vi "HFRR ADV v07 new software.vi"() -> ()   [LabVIEW 2025] (continued)
            n3590 = Concatenate Strings(w4524, w4494) -> (w4555:string)
            n3591 = Concatenate Strings(w4576, w4474, w4577, w4570) -> (w4579:string)
            n3592 = Concatenate Strings(w4526, w4521) -> (w4553:string)
            n3593 = Concatenate Strings(w4525, w4511) -> (w4552:string)
            n3594 = Concatenate Strings(w4524, w4493) -> (w4554:string)
            n3595 = Concatenate Strings(w4526, w4520) -> (w4548:string)
            n3596 = Concatenate Strings(w4525, w4510) -> (w4549:string)
            n3597 = Concatenate Strings(w4524, w4492) -> (w4547:string)
            n3598 = Concatenate Strings(w4526, w4519) -> (w4545:string)
            n3599 = Concatenate Strings(w4525, w4509) -> (w4544:string)
            n3600 = Concatenate Strings(w4524, w4491) -> (w4546:string)
            n3601 = Concatenate Strings(w4556, w4557, w4555) -> (w4558:string)
            n3602 = Concatenate Strings(w4526, w4518) -> (w4535:string)
            n3603 = Concatenate Strings(w4525, w4508) -> (w4536:string)
            n3604 = Concatenate Strings(w4526, w4517) -> (w4532:string)
            n3605 = Concatenate Strings(w4525, w4507) -> (w4531:string)
            n3606 = Concatenate Strings(w4524, w4490) -> (w4534:string)
            n3607 = Concatenate Strings(w4524, w4489) -> (w4533:string)
            n3608 = Concatenate Strings("{\"SecretKey\":\"", w4573, w4579, "\",\"UUID\" : \"", w4568, "\",\"SensorInformation\":", "[{" ("string")) -> (w4506:string)
            n3609 = Concatenate Strings(w4553, w4552, w4554) -> (w4551:string)
            n3610 = Concatenate Strings(w4548, w4549, w4547) -> (w4550:string)
            n3611 = Concatenate Strings(w4545, w4544, w4546) -> (w4543:string)
            n3612 = Concatenate Strings(w4535, w4536, w4534) -> (w4537:string)
            n3613 = Concatenate Strings(w4532, w4531, w4533) -> (w4530:string)
            n3614 = Concatenate Strings(w4529, w4541, w4558, w4499) -> (w4505:string)
            n3615 = Concatenate Strings(w4529, w4540, w4551, w4499) -> (w4504:string)
            n3616 = Concatenate Strings(w4529, w4539, w4550, w4499) -> (w4503:string)
            n3617 = Concatenate Strings(w4529, w4538, w4543, w4499) -> (w4502:string)
            n3618 = Concatenate Strings(w4529, w4528, w4537, w4499) -> (w4501:string)
            n3619 = Concatenate Strings(w4529, w4527, w4530, "\"}" ("string")) -> (w4500:string)
            n3620 = Concatenate Strings(w4506, w4505, w4504, w4503, w4502, w4501, w4500, "]}" ("string")) -> (w4497:string)
            n3621 = local read "SEN.RUN HRS"() -> (w4464:dbl)
            n3622 = disable-structure shown="Disabled" {
              frame Disabled {
                n3623 = local read "state"() -> (w4583:string[])
                n3624 = Delete From Array(array=w4583, index=0) -> (array with subset deleted=w4581:string[])  [unwired: 1 in, 1 out]
                n3625 = for {
                  N: 6 -> [_]
                  tunnel: w4581 -> [w4594] mode=indexing
                  tunnel: [w4593] -> w4580 mode=indexing
                  n3626 = Equal?(x=w4594, y="Warning") -> (x = y?=w4590:bool)
                  n3627 = Equal?(x=w4594, y="Healthy") -> (x = y?=w4587:bool)
                  n3628 = Select(t="2" ("y"), s=w4590, f="3" ("y")) -> (s? t:f=w4585:string)
                  n3629 = Select(t="1" ("y"), s=w4587, f=w4585) -> (s? t:f=w4593:string)
                }
                "state1" <- w4580
              }
              frame Enabled {
              }
            }
            n3630 = stacked-sequence {
              tunnel: w4497 -> [w4605 _ _]
              tunnel: [_ _ w4621] -> _
              frame #0 {
                (unwired) FALSE ("convert eol (F)")
                w4607 = enum16{"start", "end", "current"}."start" ("pos mode (0:2)")
                n3631 = local read "Path"() -> (w4601:path)
                n3632 = Path To String(path=w4601) -> (string=w4613:string)
                n3633 = Concatenate Strings(w4613, "\\", "Sensor File Name") -> (w4614:string)
                n3634 = local write "standard output 2"(" ") -> ()
                n3635 = String To Path(string=w4614) -> (path=w4604:path)
                n3636 = call <vilib>:"Open_Create_Replace File.vi"("advisory dialog? (display:T)"=FALSE, "function (open:0)"=T29."create or replace", "file path"=w4604) -> ("error out"=w4617:errorcluster, "refnum"=w4616:refnum<file>)  [unwired: 5 in, 2 out]
                n3637 = Set File Position(refnum=w4616, from (0:start)=w4607, error in=w4617) -> (refnum out=w4597:refnum<file>, error out=w4596:errorcluster)  [unwired: 1 in]
                n3638 = Write to Binary File(file (use dialog)=w4597, data=" ", error in=w4596, 5:FALSE ("prepend array or string size? (T)")) -> (refnum out=w4608:refnum<file>, error out=w4609:errorcluster)  [unwired: 2 in, 1 out]
                n3639 = Set File Position(offset (in bytes) (0)=w4607, refnum=w4608, error in=w4609) -> (refnum out=w4600:refnum<file>, error out=w4599:errorcluster)  [unwired: 1 in]
                n3640 = Write to Binary File(file (use dialog)=w4600, data=w4605, error in=w4599, 5:FALSE ("prepend array or string size? (T)")) -> (error out=w4603:errorcluster)  [unwired: 2 in, 2 out]
                n3641 = flat-sequence {
                  tunnel: w4604 -> [w4619]
                  tunnel: w4603 -> [_]
                  frame #0 {
                    n3642 = call <vilib>:"Read Characters From File.vi"("file path (dialog if empty)"=w4619) -> ("character string"=→"Sensor Health JSON string":string)  [unwired: 5 in, 3 out]
                  }
                }
                "SinglePoint  2" <- w4605
              }
              frame #1 {
              }
              frame #2 {
                (unwired) "\"Stored\": true" ("string")
                n3643 = call <vilib>:"System Exec.vi"("run minimized? (F)"=TRUE, "wait until completion? (T)"=TRUE, "working directory"=path "C:/LAB-IQ-NXT", "command line"="C:\\LAB-IQ-NXT\\JPostH.bat") -> ("standard error"=→"Respose From Server 2":string, "standard output"=w4624:string)  [unwired: 4 in, 2 out]
                "standard output 2" <- w4624
                n3644 = Match Pattern(string=w4624, regular expression="JSONH Check String") -> (match substring=w4622:string, offset past match=w4621:i32)  [unwired: 1 in, 2 out]
                n3645 = Equal?(x=w4622, y="JSONH Check String") -> (x = y?=→"Upload \nConfirmed 2":bool)
              }
            }
            n3646 = Divide(x=w4464, y=3600.0 ("f")) -> (x/y=w4457:dbl)
            n3647 = local read "run time"() -> (w4514:string[])
            n3648 = Round To Nearest(number=w4457) -> (nearest integer value=w4456:dbl)
            n3649 = Number To Decimal String(number=w4456) -> (decimal integer string=w4455:string)  [unwired: 1 in]
            n3650 = Index Array(array="Sensor Information", index (col) #1=0 ("disabled index (col)"), index (col) #2=1 ("index (col)"), index (col) #3=2 ("index (col)"), index (col) #4=3 ("index (col)")) -> (element #1=→"Sensor name":string[], element #2=→"model num":string[], element #3=→"run time":string[], element #4=→"state":string[])  [unwired: 4 in]
            n3651 = Insert Into Array(array=w4514, index=1, new element #1=w4455, new element #2=w4455, new element #3=w4455, new element #4=w4455, new element #5=w4455, new element #6=w4455) -> (w4479:string[])
            "run" <- w4479
            n3652 = local read "out"() -> (w4461:string[])
            n3653 = local read "Sensor Information"() -> (w4481:string[][])
            n3654 = Replace Array Subset(array=w4481, new element #1=w4479, index (col) #1=2 ("disabled index (col)"), new element #2=w4461, index (col) #2=3 ("index (col)")) -> (w4480:string[][])  [unwired: 2 in]
            n3655 = local write "Sensor Information"(w4480) -> ()
          }
        }
        n3656 = case shown="True" w4428 {
          frame False {
          }
          frame True {
            n3657 = Equal?(x="FLAG", y=0.0) -> (x = y?=w4445:bool)
            n3658 = case shown="False" w4445 {
              frame False {
                n3659 = Get Date/Time In Seconds() -> (seconds since 1Jan1904=w4451:timestamp)
                n3660 = local read "START 2"() -> (w4449:dbl)
                n3661 = To Double Precision Float(number=w4451) -> (double precision float=w4450:dbl)
                n3662 = Subtract(x=w4450, y=w4449) -> (x-y=→"SENSOR TIME  2":dbl)
              }
              frame True {
                n3663 = Get Date/Time In Seconds() -> (seconds since 1Jan1904=w4453:timestamp)
                n3664 = To Double Precision Float(number=w4453) -> (double precision float=→"START 2":dbl)
                n3665 = local write "FLAG"(100.0 ("FLAG")) -> ()
              }
            }
          }
        }
        n3666 = disable-structure shown="Disabled" {
          disable-tunnel: w4431 -> [w4440 _]
          disable-tunnel: [w4439 _] -> w4430
          frame Disabled {
            n3667 = local read "Json St Flg"() -> (w4438:bool)
            n3668 = case shown="True" w4438 {
              tunnel: w4440 -> [w4441 w4443]
              tunnel: [w4441 w4442] -> w4439
              frame False {
              }
              frame True {
                n3669 = Increment(x=w4443) -> (x+1=w4442:dbl)
                "T cycle" <- w4442
                n3670 = local write "Json St Flg"(FALSE ("Json St Flg")) -> ()
              }
            }
          }
          frame Enabled {
          }
        }
        n3671 = local read "Quit"() -> (w4425:bool)
      }
    }
    frame Enabled {
    }
  }
  n3672 = stacked-sequence {
    tunnel: [w4823] -> w38
    frame #0 {
      w4823 = FALSE ("Upload \nConfirmed")
      n3673 = local write "Upload \nConfirmed"(w4823) -> ()
      n3674 = local write "St Str"("") -> ()
    }
  }
  n3675 = disable-structure shown="Disabled" {
    disable-tunnel: w38 -> [w4824 _]
    frame Disabled {
      n3676 = case shown="True" {
        selector: _ -> [_ _]
        tunnel: w4824 -> [_ w4825]
        frame False {
        }
        frame True {
          n3677 = while {
            tunnel: [w4831] -> _
            tunnel: w4825 -> [_]
            i -> [w4831]
            stop <- w4826 stop-if-true
            n3678 = local read "Json End Flg"() -> (w4830:bool)
            n3679 = Wait (ms)(milliseconds to wait=u32 20 ("Refresh Rate (ms)")) -> ()  [unwired: 1 out]
            n3680 = local read "refresh flag"() -> (w4827:bool)
            n3681 = local read "RUN"() -> (w4828:bool)
            n3682 = And(x=w4828, y=w4827) -> (x .and. y?=w4829:bool)
            n3683 = Or(x=w4829, y=w4830) -> (x .or. y?=w4832:bool)
            "AR Led" <- w4832
            n3684 = case shown="True" w4832 {
              frame False {
              }
              frame True {
                w4849 = "\",\""
                n3685 = local read "UUID"() -> (w4847:string)
                n3686 = local write "refresh flag"(FALSE ("refresh flag")) -> ()
                n3687 = local read "time"() -> (w4836:dbl)
                n3688 = Multiply(x=w4836, y=60.0) -> (x*y=w4835:dbl)
                n3689 = Concatenate Strings("UUID\" : \"", w4847, "\"}") -> (w4850:string)
                n3690 = Number To Fractional String(number=w4835, width (-)=i16 10, precision (6)=i16 4) -> (F-format string=w4864:string)  [unwired: 1 in]
                n3691 = Concatenate Strings("{", "\"Time\":\"", w4864, w4849) -> (w4859:string)
                n3692 = stacked-sequence {
                  tunnel: w4849 -> [w4912 w4920 w4927 w4935 w4943 w4952 w4959]
                  tunnel: [w4913 _ _ _ _ _ _] -> w4863
                  tunnel: [_ w4921 _ _ _ _ _] -> w4862
                  tunnel: [_ _ w4928 _ _ _ _] -> w4861
                  tunnel: [_ _ _ w4937 _ _ _] -> w4860
                  tunnel: w4850 -> [_ _ _ _ _ _ w4970]
                  tunnel: [_ _ _ _ _ _ w4969] -> w4846
                  tunnel: [_ _ _ _ _ w4949 _] -> w4845
                  tunnel: [_ _ _ _ w4942 _ _] -> w4844
                  frame #0 {
                    n3693 = local read "NORMAL LOAD"() -> (w4911:dbl)
                    n3694 = Number To Fractional String(number=w4911, width (-)=i16 10, precision (6)=i16 4) -> (F-format string=w4914:string)  [unwired: 1 in]
                    n3695 = Concatenate Strings("NormalLoad\":\"", w4914, w4912) -> (w4913:string)
                  }
                  frame #1 {
                    n3696 = local read "Temp"() -> (w4919:dbl)
                    n3697 = Number To Fractional String(number=w4919, width (-)=i16 10, precision (6)=i16 4) -> (F-format string=w4922:string)  [unwired: 1 in]
                    n3698 = Concatenate Strings("Temperature\":\"", w4922, w4920) -> (w4921:string)
                  }
                  frame #2 {
                    n3699 = local read "cof"() -> (w4925:dbl)
                    n3700 = Number To Fractional String(number=w4925, width (-)=i16 10, precision (6)=i16 4) -> (F-format string=w4929:string)  [unwired: 1 in]
                    n3701 = Concatenate Strings("FrictionalForce\":\"", w4929, w4927) -> (w4928:string)
                  }
                  frame #3 {
                    n3702 = local read "Set Hz"() -> (w4933:dbl)
                    n3703 = Multiply(x=w4933, y=60.0) -> (x*y=w4932:dbl)
                    n3704 = Number To Fractional String(number=w4932, width (-)=i16 10, precision (6)=i16 4) -> (F-format string=w4938:string)  [unwired: 1 in]
                    n3705 = Concatenate Strings("Speed\":\"", w4938, w4935) -> (w4937:string)
                  }
                  frame #4 {
                    n3706 = local read item#-1() -> (w4941)
                    n3707 = Number To Fractional String(number=w4941, width (-)=i16 10, precision (6)=i16 4) -> (F-format string=w4945:string)  [unwired: 1 in]
                    n3708 = Concatenate Strings("LinearDeformation\":\"", w4945, w4943) -> (w4942:string)
                  }
                  frame #5 {
                    n3709 = local read "AIR TEMP"() -> (w4948:dbl)
                    n3710 = local read "Json St Flg"() -> (w4950:bool)
                    n3711 = local read "Json End Flg"() -> (w4951:bool)
                    n3712 = Number To Fractional String(number=w4948, width (-)=i16 10, precision (6)=i16 4) -> (F-format string=w4954:string)  [unwired: 1 in]
                    n3713 = Concatenate Strings("Vibration\":\"", w4954, w4952) -> (w4949:string)
                    n3714 = And(x=w4950, y=w4951) -> ()  [unwired: 1 out]
                  }
                  frame #6 {
                    n3715 = local read "Json End Flg"() -> (w4958:bool)
                    n3716 = Get Date/Time In Seconds() -> (seconds since 1Jan1904=w4966:timestamp)
                    n3717 = local read "Json St Flg"() -> (w4957:bool)
                    n3718 = To Double Precision Float(number=w4966) -> (double precision float=w4965:dbl)
                    n3719 = Subtract(x=w4965, y=2082844800.0) -> (x-y=w4963:dbl)
                    n3720 = Number To Fractional String(number=w4963, width (-)=i16 12, precision (6)=i16 0) -> (F-format string=w4960:string)  [unwired: 1 in]
                    n3721 = case shown="True" w4958 {
                      tunnel: ["" w4973] -> w4967
                      tunnel: w4960 -> [_ w4974]
                      tunnel: w4959 -> [_ w4972]
                      frame False {
                      }
                      frame True {
                        n3722 = local write "Json End Flg"(FALSE ("Json St Flg")) -> ()
                        n3723 = Concatenate Strings("End\": \"", w4974, w4972) -> (w4973:string)
                      }
                    }
                    n3724 = case shown="True" w4957 {
                      tunnel: [w4977 w4980] -> w4968
                      tunnel: w4960 -> [_ w4981]
                      tunnel: w4959 -> [_ w4978]
                      frame False {
                        n3725 = local read "St Str"() -> (w4977:string)
                      }
                      frame True {
                        n3726 = Concatenate Strings("Start\":\"", w4981, w4978) -> (w4980:string)
                        "St Str" <- w4980
                        n3727 = local write "Json St Flg"(FALSE ("Json St Flg")) -> ()
                      }
                    }
                    n3728 = Concatenate Strings(w4968, w4967, w4970) -> (w4969:string)
                  }
                }
                n3729 = local read "FILE"() -> (w4838:string)
                n3730 = Concatenate Strings("\",\"OperatorID\":\"" ("string"), "Operator ID") -> (w4841:string)
                n3731 = Concatenate Strings("\",\"DatasetTitle\":\"" ("string"), w4838) -> (w4840:string)
                n3732 = Concatenate Strings("\",\"SerialNumber\":\"" ("string"), "Serial No") -> (w4870:string)
                n3733 = Concatenate Strings("\",\"ModelNumber\":\"" ("string"), "Model No") -> (w4869:string)
                n3734 = Concatenate Strings(w4870, w4869) -> (w4852:string)
                n3735 = Concatenate Strings("{\"SecretKey\":\"", "Secret Key", w4852, w4841, w4840, "\",\"Samples\":[") -> (w4857:string)
                n3736 = Concatenate Strings(w4859, w4863, w4862, w4861, w4860, w4844, w4845, w4846) -> (w4858:string)
                n3737 = Concatenate Strings(w4857, w4858, "]}") -> (w4856:string)
                n3738 = stacked-sequence {
                  tunnel: w4856 -> [w4885 _ _]
                  tunnel: [_ _ w4902] -> _
                  frame #0 {
                    (unwired) FALSE ("convert eol (F)")
                    w4887 = enum16{"start", "end", "current"}."start" ("pos mode (0:2)")
                    n3739 = Path To String(path="Path") -> (string=w4893:string)
                    n3740 = Concatenate Strings(w4893, "\\", "Data File Name") -> (w4895:string)
                    n3741 = local write "standard output"(" ") -> ()
                    n3742 = String To Path(string=w4895) -> (path=w4884:path)
                    n3743 = call <vilib>:"Open_Create_Replace File.vi"("advisory dialog? (display:T)"=FALSE, "function (open:0)"=T29."create or replace", "file path"=w4884) -> ("error out"=w4898:errorcluster, "refnum"=w4897:refnum<file>)  [unwired: 5 in, 2 out]
                    n3744 = Set File Position(refnum=w4897, from (0:start)=w4887, error in=w4898) -> (refnum out=w4878:refnum<file>, error out=w4877:errorcluster)  [unwired: 1 in]
                    n3745 = Write to Binary File(file (use dialog)=w4878, data=" ", error in=w4877, 5:FALSE ("prepend array or string size? (T)")) -> (refnum out=w4888:refnum<file>, error out=w4889:errorcluster)  [unwired: 2 in, 1 out]
                    n3746 = Set File Position(offset (in bytes) (0)=w4887, refnum=w4888, error in=w4889) -> (refnum out=w4881:refnum<file>, error out=w4880:errorcluster)  [unwired: 1 in]
                    n3747 = Write to Binary File(file (use dialog)=w4881, data=w4885, error in=w4880, 5:FALSE ("prepend array or string size? (T)")) -> (error out=w4883:errorcluster)  [unwired: 2 in, 2 out]
                    n3748 = flat-sequence {
                      tunnel: w4884 -> [w4900]
                      tunnel: w4883 -> [_]
                      frame #0 {
                        n3749 = call <vilib>:"Read Characters From File.vi"("file path (dialog if empty)"=w4900) -> ("character string"=→"JSON string":string)  [unwired: 5 in, 3 out]
                      }
                    }
                    "SinglePoint" <- w4885
                  }
                  frame #1 {
                  }
                  frame #2 {
                    (unwired) "\"Stored\": true" ("string")
                    n3750 = call <vilib>:"System Exec.vi"("run minimized? (F)"=TRUE, "wait until completion? (T)"=TRUE, "working directory"=path "C:/LAB-IQ-NXT", "command line"="C:\\LAB-IQ-NXT\\JPost.bat") -> ("standard error"=→"Respose From Server":string, "standard output"=w4905:string)  [unwired: 4 in, 2 out]
                    "standard output" <- w4905
                    n3751 = Match Pattern(string=w4905, regular expression="JSON Check String") -> (match substring=w4903:string, offset past match=w4902:i32)  [unwired: 1 in, 2 out]
                    n3752 = Equal?(x=w4903, y="JSON Check String") -> (x = y?=→"Upload \nConfirmed":bool)
                  }
                }
              }
            }
            n3753 = local read "Quit"() -> (w4826:bool)
          }
        }
      }
    }
    frame Enabled {
    }
  }
  n3754 = disable-structure shown="Disabled" {
    disable-tunnel: _ -> [w4988 _]
    frame Disabled {
      n3755 = while {
        shift-right: [w4996] -> w4984
        shift-left: _ -> [w4997]
        shift-right: [w4994] -> w4985
        shift-left: errorcluster {"status"=TRUE, "code"=0, "source"="Init"} ("error out") -> [w4995]
        shift-right: [w4992] -> _
        shift-left: "" -> [w4993]
        tunnel: [w4990] -> _
        tunnel: w4988 -> [_]
        i -> [w4990]
        stop <- w4989 stop-if-true
        n3756 = flat-sequence {
          tunnel: [w4998] -> w4991
          frame #0 {
            n3757 = Wait (ms)(milliseconds to wait=10.0 ("Delay")) -> (millisecond timer value=w4998:u32)
          }
        }
        n3758 = case shown="No Error" w4995 {
          selector: w4995 -> [w5028 w5147]
          tunnel: [w5011 w5149] -> w4996
          tunnel: [w5010 w5148] -> w4994
          tunnel: w4997 -> [w5029 w5141]
          tunnel: w4993 -> [w5009 w5140]
          tunnel: [w5008 w5140] -> w4992
          tunnel: w4991 -> [_ _]
          frame No Error {
            n3759 = Concatenate Strings("\r", "\n") -> (w5020:string)  [unwired: 1 in]
            n3760 = case shown="True" w5021 {
              tunnel: w5029 -> [w5053 w5060]
              tunnel: w5028 -> [w5052 w5059]
              tunnel: [w5053 w5058] -> w5027
              tunnel: [w5052 w5057] -> w5007
              tunnel: w5020 -> [_ w5056]
              frame False {
              }
              frame True {
                n3761 = VISA Write(VISA resource name=w5060, write buffer=w5056, error in (no error)=w5059) -> (VISA resource name out=w5058:refnum<visa-resource-name>, error out=w5057:errorcluster)  [unwired: 1 out]
                n3762 = local write "Read String"("") -> ()
                n3763 = local write item#-1(FALSE) -> ()
              }
            }
            n3764 = property class="Instr"(reference=w5027, error in=w5007) -> (reference out=w5026:refnum<visa-resource-name>, error out=w5025:errorcluster, "Serial Settings:Number of Bytes at Serial Port"=w5024:u32)
            n3765 = Greater?(x=w5024, y=u32 100) -> (0:w5022:bool)
            n3766 = case shown="True" w5022 {
              tunnel: w5026 -> [w5063 w5087]
              tunnel: w5025 -> [w5062 w5086]
              tunnel: w5024 -> [_ w5085]
              tunnel: [w5063 w5084] -> w5013
              tunnel: [w5062 w5083] -> w5012
              tunnel: w5009 -> [w5061 w5082]
              tunnel: [w5061 ""] -> w5008
              frame False {
              }
              frame True {
                w5072 = u32 6 ("y")
                # "Page 84 of \nmanual"
                n3767 = VISA Read(VISA resource name=w5087, byte count=w5085, error in (no error)=w5086) -> (VISA resource name out=w5084:refnum<visa-resource-name>, read buffer=w5080:string, error out=w5083:errorcluster)  [unwired: 1 out]
                n3768 = while {
                  tunnel: w5080 -> [w5136]
                  tunnel: [w5132] -> w5074 mode=indexing
                  tunnel: [w5126] -> w5078 mode=indexing
                  tunnel: [w5124] -> _
                  i -> [w5124]
                  stop <- w5129 stop-if-true
                  n3769 = String Subset(string=w5136, offset (0)=w5124) -> (substring=w5131:string)  [unwired: 1 in]
                  n3770 = String To Byte Array(string=w5131) -> (unsigned byte array=w5135:u8[])
                  n3771 = String Length(string=w5131) -> (length=w5130:i32)
                  n3772 = Index Array(array=w5135) -> (element=w5134:u8)  [unwired: 1 in]
                  n3773 = Equal To 0?(x=w5130) -> (x = 0?=w5129:bool)
                  n3774 = Number To Boolean Array(number=w5134) -> (Boolean array=w5128:bool[])
                  n3775 = Reverse 1D Array(array=w5128) -> (reversed array=w5127:bool[])
                  n3776 = And(x=w5128, y=bool[] [FALSE, FALSE, FALSE, FALSE, FALSE, FALSE, TRUE, TRUE] ("Boolean array")) -> (x .and. y?=w5132:bool[])
                  n3777 = And(x=w5127, y=bool[] [FALSE, FALSE, TRUE, TRUE, TRUE, TRUE, TRUE, TRUE] ("Boolean array")) -> (x .and. y?=w5126:bool[])
                }
                n3778 = Concatenate Strings(w5082, w5080) -> (→"Read String":string)
                n3779 = while {
                  tunnel: w5074 -> [w5123] mode=indexing
                  tunnel: [w5119] -> w5077
                  i -> [w5119]
                  stop <- w5120 stop-if-true
                  n3780 = Search 1D Array(1D array=w5123, element=TRUE) -> (index of element=w5121:i32)  [unwired: 1 in]
                  n3781 = Less Than 0?(x=w5121) -> (x < 0?=w5120:bool)
                }
                n3782 = Delete From Array(array=w5078, length=w5077, index (row)=0) -> (array with subset deleted=w5073:bool[][])  [unwired: 1 in, 1 out]
                n3783 = Array Size(array=w5073) -> (size(s)=w5075:i32[])
                n3784 = Index Array(array=w5075) -> (element=w5067:i32)  [unwired: 1 in]
                n3785 = Greater?(x=w5067, y=w5072) -> (0:w5070:bool)
                n3786 = Subtract(x=w5067, y=w5072) -> (x-y=w5071:u32)
                n3787 = Select(t=w5071, s=w5070, f=u32 0) -> (s? t:f=w5068:u32)
                n3788 = while {
                  tunnel: w5073 -> [w5106]
                  tunnel: [w5108] -> w5066 mode=indexing
                  tunnel: w5068 -> [w5090]
                  i -> [w5107]
                  stop <- w5105 stop-if-true
                  w5097 = 6 ("index")
                  w5096 = 2 ("length")
                  # "Page 65 of \nmanual"
                  n3789 = Multiply(x=u32 3 ("y"), y=w5107) -> (x*y=w5104:u32)
                  n3790 = Divide(x=u32 102 ("y"), y=u32 65520) -> (x/y=w5114:dbl)
                  n3791 = Greater Or Equal?(x=w5104, y=w5090) -> (x >= y?=w5105:bool)
                  n3792 = Index Array(array=w5106, index (row) #1=w5104) -> (element #1=w5102:bool[], element #2=w5101:bool[], element #3=w5100:bool[])  [unwired: 5 in]
                  n3793 = Reverse 1D Array(array=w5102) -> (reversed array=w5095:bool[])
                  n3794 = Reverse 1D Array(array=w5101) -> (reversed array=w5099:bool[])
                  n3795 = Reverse 1D Array(array=w5100) -> (reversed array=w5098:bool[])
                  n3796 = Delete From Array(array=w5095, length=w5096, index=w5097) -> (array with subset deleted=w5091:bool[])  [unwired: 1 out]
                  n3797 = Delete From Array(array=w5099, length=w5096, index=w5097) -> (array with subset deleted=w5092:bool[])  [unwired: 1 out]
                  n3798 = Delete From Array(array=w5098, length=w5096, index=w5097) -> (array with subset deleted=w5093:bool[])  [unwired: 1 out]
                  n3799 = Insert Into Array(array=bool[] [] ("Boolean array"), new element #1=w5091, new element #2=w5092, new element #3=w5093) -> (w5094:bool[])  [unwired: 1 in]
                  n3800 = Boolean Array To Number(Boolean array=w5094) -> (number=w5103:u32)
                  n3801 = Multiply(x=w5114, y=w5103) -> (x*y=w5113:dbl)
                  n3802 = Decrement(x=w5113) -> (x-1=w5112:dbl)
                  n3803 = Divide(x=w5112, y=u32 100) -> (x/y=w5110:dbl)
                  n3804 = Multiply(x=w5110, y=u32 10) -> (x*y=w5108:dbl)
                }
                n3805 = Delete From Array(array=w5066) -> (array with subset deleted=w5065:dbl[])  [unwired: 2 in, 1 out]
                "Waveform Graph 5" <- w5065
                "Waveform Chart 3" <- w5065
                n3806 = call-poly <vilib>:"Mean.vi"("X"=w5065) -> ("mean"=w5064:dbl)  [unwired: 1 out]
                n3807 = case shown="True" {
                  selector: _ -> [_ _]
                  tunnel: w5064 -> [_ w5089]
                  frame False {
                  }
                  frame True {
                    n3808 = local write item#-1(FALSE ("Zero 4")) -> ()
                    "z_measure" <- w5089
                  }
                }
              }
            }
            n3809 = local read item#-1() -> (w5004)
            n3810 = local read item#-1() -> (w5003)
            n3811 = local read item#-1() -> (w5005)
            n3812 = local read item#-1() -> (w5002)
            n3813 = case shown="True" w5000 {
              tunnel: w5004 -> [_ w5032]
              tunnel: w5005 -> [_ w5031]
              frame False {
              }
              frame True {
                n3814 = Build Array(w5032, w5031) -> (w5030:void[])
                n3815 = local read item#-1() -> (w5035)
                n3816 = Build Array (concatenate)(w5035, w5030) -> (w5033:void[])
                n3817 = local write item#-1(w5033) -> ()
                n3818 = local write item#-1(FALSE ("Boolean 8")) -> ()
              }
            }
            n3819 = call "Build XY Graph"("Enable"=w5002, "Reset"=w5003, "Y Input"=w5005, "X Input"=w5004) -> ("XY Graph"=w5001:cluster{"Y":dbl[], "Y":dbl[]}[])  [unwired: 6 in, 1 out]
            n3820 = case shown="True" {
              selector: _ -> [_ _]
              frame False {
              }
              frame True {
                n3821 = local read item#-1() -> (w5036)
                n3822 = Index Array(array=w5036, index (col) #1=0 ("disabled index (col)"), index (col) #2=1 ("index (col)")) -> (element #1=w5038, element #2=w5037)  [unwired: 2 in]
                n3823 = call <vilib>:"Linear Fit.vi"("Y"=w5038, "X"=w5037) -> ()  [unwired: 9 in, 5 out]
                n3824 = local write item#-1(FALSE ("Boolean 9")) -> ()
              }
            }
            n3825 = case shown="True" {
              selector: _ -> [_ _]
              frame False {
              }
              frame True {
                n3826 = local write item#-1(dbl[][] [] ("Captured Values")) -> ()
                n3827 = local write item#-1(FALSE ("Boolean 7")) -> ()
              }
            }
            n3828 = Concatenate Strings("\r", "\n") -> (w5015:string, w5014:string)
            n3829 = case shown="True" w5006 {
              tunnel: w5013 -> [w5045 w5051]
              tunnel: w5012 -> [w5044 w5050]
              tunnel: [w5045 w5049] -> w5011
              tunnel: [w5044 w5048] -> w5010
              tunnel: w5015 -> [_ w5047]
              frame False {
              }
              frame True {
                n3830 = VISA Write(VISA resource name=w5051, write buffer=w5047, error in (no error)=w5050) -> (VISA resource name out=w5049:refnum<visa-resource-name>, error out=w5048:errorcluster)  [unwired: 1 out]
                n3831 = local write item#-1(FALSE ("WRITE")) -> ()
              }
            }
          }
          frame Error {
            w5139 = u16 10 items=["1.0"=10, "1.5"=15, "2.0"=20] ("stop bits (10: 1 bit)")
            n3832 = Wait (ms)(milliseconds to wait=u32 20) -> ()  [unwired: 1 out]
            n3833 = VISA Close(VISA resource name=w5141, error in (no error)=w5147) -> (error out=w5146:errorcluster)
            n3834 = call <vilib>:"Clear Errors.vi"("error in (no error)"=w5146) -> ("error out"=w5145:errorcluster)  [unwired: 5 in, 1 out]
            n3835 = call-poly "VISA Configure Serial Port"("timeout (10sec)"=u32 200, "Enable Termination\nChar (T)"=TRUE ("Enable Termination\nChar (T)"), "baud rate (9600)"=u32 921600, "error in (no error)"=w5145, "stop bits (10: 1 bit)"=w5139) -> ("VISA resource name"=w5137:refnum<visa-resource-name>, "VISA resource name out"=w5149:refnum<visa-resource-name>, "error out"=w5148:errorcluster)  [unwired: 8 in]
          }
        }
        n3836 = local read "Quit"() -> (w4989:bool)
      }
      n3837 = VISA Close(VISA resource name=w4984, error in (no error)=w4985) -> (error out=w4983:errorcluster)
      n3838 = call <vilib>:"Clear Errors.vi"("error in (no error)"=w4983) -> ()  [unwired: 5 in, 2 out]
    }
    frame Enabled {
    }
  }
  n3839 = disable-structure shown="Disabled" {
    disable-tunnel: _ -> [w5154 _]
    frame Disabled {
      n3840 = while {
        tunnel: [w5161] -> _
        shift-right: [w5158] -> w5151
        shift-left: _ -> [w5160]
        shift-right: [w5159] -> w5152
        shift-left: errorcluster {"status"=TRUE, "code"=0, "source"="Init"} ("error out") -> [w5157]
        tunnel: w5154 -> [_]
        i -> [w5161]
        stop <- w5155 stop-if-true
        n3841 = flat-sequence {
          tunnel: w5157 -> [w5252]
          tunnel: [w5252] -> w5156
          frame #0 {
            n3842 = Wait (ms)(milliseconds to wait=u32 50) -> ()  [unwired: 1 out]
          }
        }
        n3843 = case shown="No Error" w5156 {
          selector: w5156 -> [w5202 w5245]
          tunnel: w5160 -> [w5201 w5244]
          tunnel: [w5168 w5235] -> w5159
          tunnel: [w5169 w5243] -> w5158
          frame No Error {
            w5195 = T30 {"Mode"=enum."RTU", "Slave Address"=1} ("Serial Parameters")
            n3844 = call-poly <vilib>:"MB Serial Master Query (poly).vi"("VISA resource name"=w5201, "Starting Address"=i16 1000, "Quantity"=u16 1, "Timeout"=u32 1000, "error in"=w5202, "Serial Parameters"=w5195) -> ("VISA resource name out"=w5196:refnum<visa-resource-name>, "Input Registers"=w5198:u16[], "error out"=w5194:errorcluster)  [unwired: 10 in, 1 out]
            n3845 = Random Number (0-1)() -> (number: 0 to 1=w5183:dbl)
            n3846 = Index Array(array=w5198, index=0) -> (element=w5193:u16)
            n3847 = Subtract(x=w5183, y=0.5) -> (x-y=w5182:dbl)
            n3848 = Divide(x=w5193, y=10 ("index")) -> (x/y=w5187:dbl)
            n3849 = Multiply(x=w5182, y=0.5) -> (x*y=w5181:dbl)
            n3850 = Add(x=w5187, y=w5181) -> (x+y=w5186:dbl)
            n3851 = local read "Amb temp"() -> (w5170:dbl)
            n3852 = Multiply(x=w5186, y=0.2) -> (x*y=w5190:dbl)
            n3853 = Multiply(x=w5170, y=0.8) -> (x*y=w5188:dbl)
            n3854 = Add(x=w5190, y=w5188) -> (x+y=w5171:dbl)
            n3855 = local read "set temp old"() -> (w5165:dbl)
            n3856 = local write "Amb temp"(w5171) -> ()
            n3857 = Select(t="SetTemp 2", s="Heater", f=100.0) -> (s? t:f=w5166:dbl)
            n3858 = Not Equal?(x=w5166, y=w5165) -> (x != y?=w5164:bool)
            n3859 = case shown="True" w5164 {
              tunnel: w5196 -> [w5230 w5232]
              tunnel: [w5229 w5232] -> w5176
              tunnel: w5194 -> [w5228 w5231]
              tunnel: [w5227 w5231] -> w5174
              tunnel: w5166 -> [w5222 _]
              tunnel: w5195 -> [w5224 w5233]
              tunnel: [w5224 w5233] -> w5177
              frame True {
                n3860 = Multiply(x=w5222, y=10 ("index")) -> (x*y=w5221:dbl)
                n3861 = call-poly <vilib>:"MB Serial Master Query (poly).vi"("VISA resource name"=w5230, "Address"=u16 0, "Holding Register"=w5221, "Timeout"=u32 1000, "error in"=w5228, "Serial Parameters"=w5224) -> ("VISA resource name out"=w5229:refnum<visa-resource-name>, "error out"=w5227:errorcluster)  [unwired: 11 in, 1 out]
                "set temp old" <- w5222
              }
              frame False {
              }
            }
            n3862 = flat-sequence {
              tunnel: [w5203] -> _
              tunnel: [w5203] -> w5173
              tunnel: w5174 -> [w5203]
              frame #0 {
                n3863 = Wait (ms)(milliseconds to wait=u32 100) -> ()  [unwired: 1 out]
              }
            }
            n3864 = call "Elapsed Time12"("Time Target (s)"=2.0, "Auto Reset"=TRUE) -> ("Time has Elapsed"=w5178:bool)  [unwired: 10 in, 7 out]
            n3865 = case shown="True" w5178 {
              tunnel: w5177 -> [w5207 w5220]
              tunnel: [w5207 w5220] -> _
              tunnel: [w5206 w5218] -> w5169
              tunnel: w5176 -> [w5206 w5219]
              tunnel: [w5205 w5216] -> w5168
              tunnel: w5173 -> [w5205 w5217]
              frame False {
              }
              frame True {
                n3866 = call-poly <vilib>:"MB Serial Master Query (poly).vi"("VISA resource name"=w5219, "Starting Address"=i16 1003 ("Addr"), "Quantity"=u16 1, "Timeout"=u32 1000, "error in"=w5217, "Serial Parameters"=w5220) -> ("VISA resource name out"=w5218:refnum<visa-resource-name>, "Input Registers"=w5213:u16[], "error out"=w5216:errorcluster)  [unwired: 10 in, 1 out]
                n3867 = Index Array(array=w5213, index=0) -> (element=w5212:u16)
                n3868 = Divide(x=w5212, y=u16 10) -> (x/y=w5208:dbl)
                n3869 = local write "set temp old"(w5208) -> ()
                n3870 = local write "SetTemp"(w5208) -> ()
              }
            }
            "Error Code" <- w5168
            n3871 = Unbundle(w5168) -> ("status"=→"TK4 status":bool)  [unwired: 2 out]
            "SetTemp" <- "SetTemp 2"
          }
          frame Error {
            w5247 = u16 0 items=["None", "Odd", "Even", "Mark", "Space"] ("Parity")
            w5248 = u16 0 items=["None", "XON/XOFF", "RTS/CTS", "XON/XOFF & RTS/CTS", "DTR/DSR", "XON/XOFF & DTR/DSR"] ("Flow Control")
            n3872 = VISA Clear(VISA resource name=w5244, error in (no error)=w5245) -> (VISA resource name out=w5238:refnum<visa-resource-name>, error out=w5236:errorcluster)
            n3873 = VISA Close(VISA resource name=w5238, error in (no error)=w5236) -> (error out=w5237:errorcluster)
            n3874 = call <vilib>:"Clear Errors.vi"("error in (no error)"=w5237) -> ("error out"=w5246:errorcluster)  [unwired: 5 in, 1 out]
            n3875 = Unbundle By Name(T30 {"Mode"=enum."RTU", "Slave Address"=1} ("input cluster")) -> ("Mode"=w5249:enum16{"RTU", "ASCII"})
            n3876 = call <vilib>:"MB Serial Init.vi"("Timeout"=u32 100, "Flow Control"=w5248, "Mode"=w5249, "error in (no error)"=w5246, "Parity"=w5247, "Baud Rate"=u32 9600, "VISA resource name"="Lubrication System COM Port :") -> ("error out"=w5235:errorcluster, "VISA resource name out"=w5243:refnum<visa-resource-name>)  [unwired: 3 in]
            n3877 = local write "set temp old"(0.0 ("set temp old")) -> ()
            n3878 = Unbundle(w5235) -> ("status"=w5234:bool)  [unwired: 2 out]
            n3879 = case shown="True" w5234 {
              selector: w5234 -> [_ w5251]
              frame False {
              }
              frame True {
                n3880 = local write "TK4 status"(w5251) -> ()
              }
            }
          }
        }
        n3881 = local read "Quit"() -> (w5155:bool)
      }
      n3882 = VISA Close(VISA resource name=w5151, error in (no error)=w5152) -> (error out=w5150:errorcluster)
      n3883 = call <vilib>:"Clear Errors.vi"("error in (no error)"=w5150) -> ()  [unwired: 5 in, 2 out]
    }
    frame Enabled {
    }
  }
